vi "Blank Module Data (Constant).vi"() -> (0 "Blank Module Data":T1)   [LabVIEW 2022 SP3]
doc: "Outputs a \"blank\" Module Data cluster. Use this to initialise the Module Data, or to reset or clear it.\n\n\"blank\" is used to mean default, empty or initial values."
uses:
  Module Data.ctl
panel:
  # "Development\ncontrols/indicators useful for development and testing, but which are not outputs of the VI"
  # "Input\nInputs to the VI"
  # "Output\nOutputs of the VI"
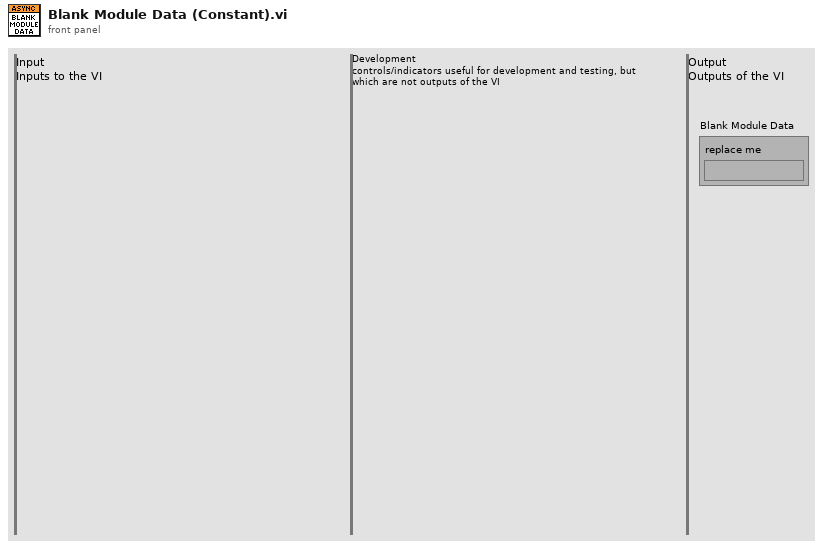
[diagram p1: front panel]
types:
  T1 = typedef "Module Data.ctl" = cluster{"replace me":string}
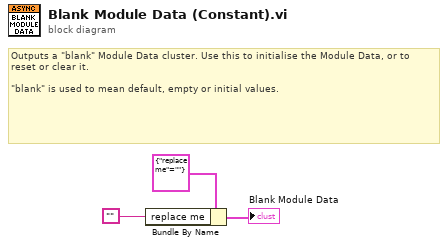
[diagram p0: block diagram]
diagram:
  # "Outputs a \"blank\" Module Data cluster. Use this to initialise the Module Data, or to reset or clear it.\n\n\"blank\" is used to mean default, empty or initial values."
  n1 = Bundle By Name(cluster=T1 {"replace me"=""} ("Module Data"), "replace me"="") -> (→"Blank Module Data":T1)
